vi "Step1_Touch.vi"   [LabVIEW 2012]
uses:
  <vilib>/NXT/Subs/MotorOutput.ctl
  <vilib>/NXT/Block Support/NXT_InputPort.ctl
types:
  T1 = typedef "NXT_InputPort.ctl" = u32
  T2 = typedef "MotorOutput.ctl" = u8
  T3 = typedef "LVHSConnector.ctl" = refnum<class "BrickReference.lvclass">
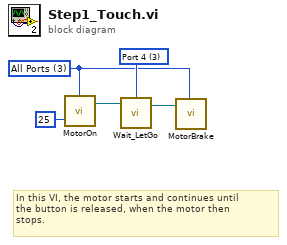
[diagram p0: block diagram]
diagram:
  w4 = T1 3 items=["Port 1", "Port 2", "Port 3", "Port 4"] ("Port (Port 1)")
  w2 = T2 3 items=["Port A"=0, "Port B"=1, "Port C"=2, "Ports A & B"=4, "Ports A & C"=5, "Ports B & C"=6, "All Ports"=3] ("Output Port (All Ports)")
  # "In this VI, the motor starts and continues until\nthe button is released, when the motor then \nstops."
  n1 = call <vilib>:"MotorOn.vi"("Power (75)"=25, "Output Port (All Ports)"=w2) -> ("NXT/EV3"=w5:T3)  [unwired: 2 in]
  n2 = call <vilib>:"Wait_LetGo.vi"("NXT/EV3"=w5, "Port (Port 1)"=w4) -> ("NXTEV3"=w3:T3)  [unwired: 2 in]
  n3 = call <vilib>:"MotorBrake.vi"("NXT/EV3"=w3, "Port (All Ports)"=w2) -> ()  [unwired: 2 in, 1 out]
